vi "lightening arrange.vi"() -> ()   [LabVIEW 2014]
panel:
  in  "panel":T1
  out "result":dbl
  out "result 2":dbl
  out "Total elecFee":dbl
  out "Group 1":bool[](array[boolean])
  out "Group 2":bool[](array[boolean])
  out "Group 3":bool[](array[boolean])
  out "NO.":i32
  out "Waveform Graph 2":dbl[][](graph)
  out "Waveform Graph":dbl[](graph)
  out "size(s)":i32
  in  "group 3 power consume (W)":dbl format="%#_13g"
  in  "group 3 Lightening period":i32
  in  "group 2 power consume (W)":dbl format="%#_13g"
  in  "group 2 Lightening period":i32
  in  "group 1 power consume (W)":dbl format="%#_13g"
  in  "group 1 Lightening period":i32
  in  "input envTemp. & elecFee":cluster{"Temp.":dbl[], "elecFee":dbl[]}={"Temp."=[29.6, 26.5, 26.8, 26.8, 26.5, 26.9, 27.8, 28.5, 26.3, 30.1, 33.3, 33.4, 33.9, 32.2, 32.7, 32.7, 32.4, 31.5, 30.5, 29.7, 28.3, 28.2, 27.9, 27.5], "elecFee"=[2.2, 2.2, 2.2, 2.2, 2.2, 2.2, 2.2, 2.2, 3.5, 3.5, 3.5, 3.5, 3.5, 3.5, 3.5, 3.5, 3.5, 3.5, 3.5, 3.5, 3.5, 3.5, 2.2, 2.2]}
  in  "input Parameter":T2={"input COP of ACs"=3.0, "input setDay Temp"=22.0, "input setNight Temp."=20.0}
  # "0~1"
  # "1~2"
  # "2~3"
  # "3~4"
  # "4~5"
  # "5~6"
  # "6~7"
  # "7~8"
  # "8~98~9"
  # "9~10"
  # "10~11"
  # "11~12"
  # "12~13"
  # "13~14"
  # "14~15"
  # "15~16"
  # "16~17"
  # "17~18"
  # "18~19"
  # "19~20"
  # "21~21"
  # "21~22"
  # "22~23"
  # "23~24"
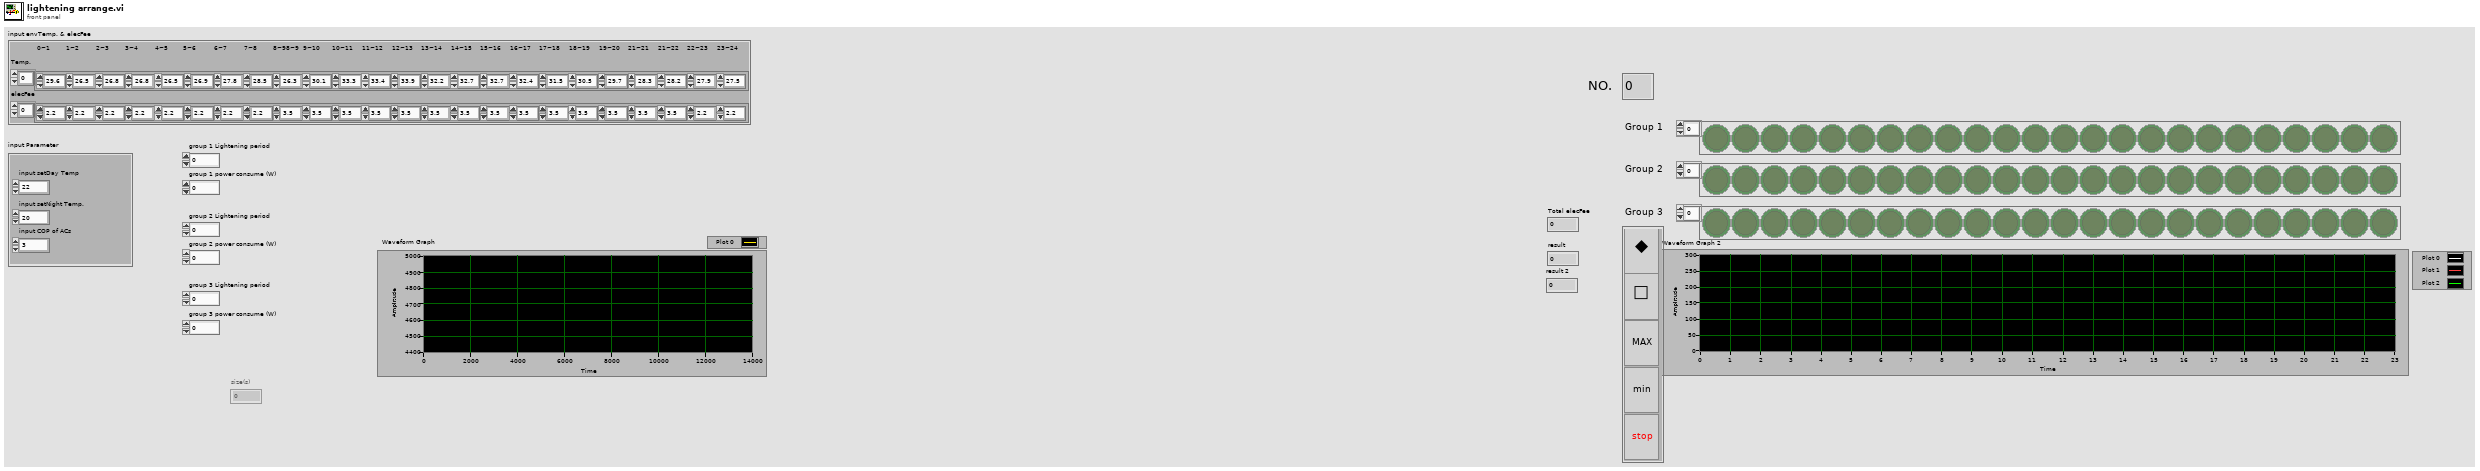
[diagram p1: front panel]
types:
  T1 = cluster{"◆":bool, "□":bool, "MAX":bool, "min":bool, "stop":bool}
  T2 = cluster{"input COP of ACs":dbl, "input setDay Temp":dbl, "input setNight Temp.":dbl}
  T3 = cluster{"group Outcome":cluster{"Lightening Schedule":bool[], "group hourly total elecFee":dbl[], "group Total elecFee":dbl, "group hourly ACs elecFee":dbl[], "group ACs elecFee":dbl, "group hourly LEDs elecFee":dbl[], "group Total LEDs elecFee":dbl}, "group Outcome 2":cluster{"Lightening Schedule":bool[], "group hourly total elecFee":dbl[], "group Total elecFee":dbl, "group hourly ACs elecFee":dbl[], "group ACs elecFee":dbl, "group hourly LEDs elecFee":dbl[], "group Total LEDs elecFee":dbl}, "group Outcome 3":cluster{"Lightening Schedule":bool[], "group hourly total elecFee":dbl[], "group Total elecFee":dbl, "group hourly ACs elecFee":dbl[], "group ACs elecFee":dbl, "group hourly LEDs elecFee":dbl[], "group Total LEDs elecFee":dbl}, "Total elecFee":dbl}[]
  T4 = cluster{"group Outcome":cluster{"Lightening Schedule":bool[], "group hourly total elecFee":dbl[], "group Total elecFee":dbl, "group hourly ACs elecFee":dbl[], "group ACs elecFee":dbl, "group hourly LEDs elecFee":dbl[], "group Total LEDs elecFee":dbl}, "group Outcome 2":cluster{"Lightening Schedule":bool[], "group hourly total elecFee":dbl[], "group Total elecFee":dbl, "group hourly ACs elecFee":dbl[], "group ACs elecFee":dbl, "group hourly LEDs elecFee":dbl[], "group Total LEDs elecFee":dbl}, "group Outcome 3":cluster{"Lightening Schedule":bool[], "group hourly total elecFee":dbl[], "group Total elecFee":dbl, "group hourly ACs elecFee":dbl[], "group ACs elecFee":dbl, "group hourly LEDs elecFee":dbl[], "group Total LEDs elecFee":dbl}, "Total elecFee":dbl}
  T5 = cluster{"Lightening Schedule":bool[], "group hourly total elecFee":dbl[], "group Total elecFee":dbl, "group hourly ACs elecFee":dbl[], "group ACs elecFee":dbl, "group hourly LEDs elecFee":dbl[], "group Total LEDs elecFee":dbl}
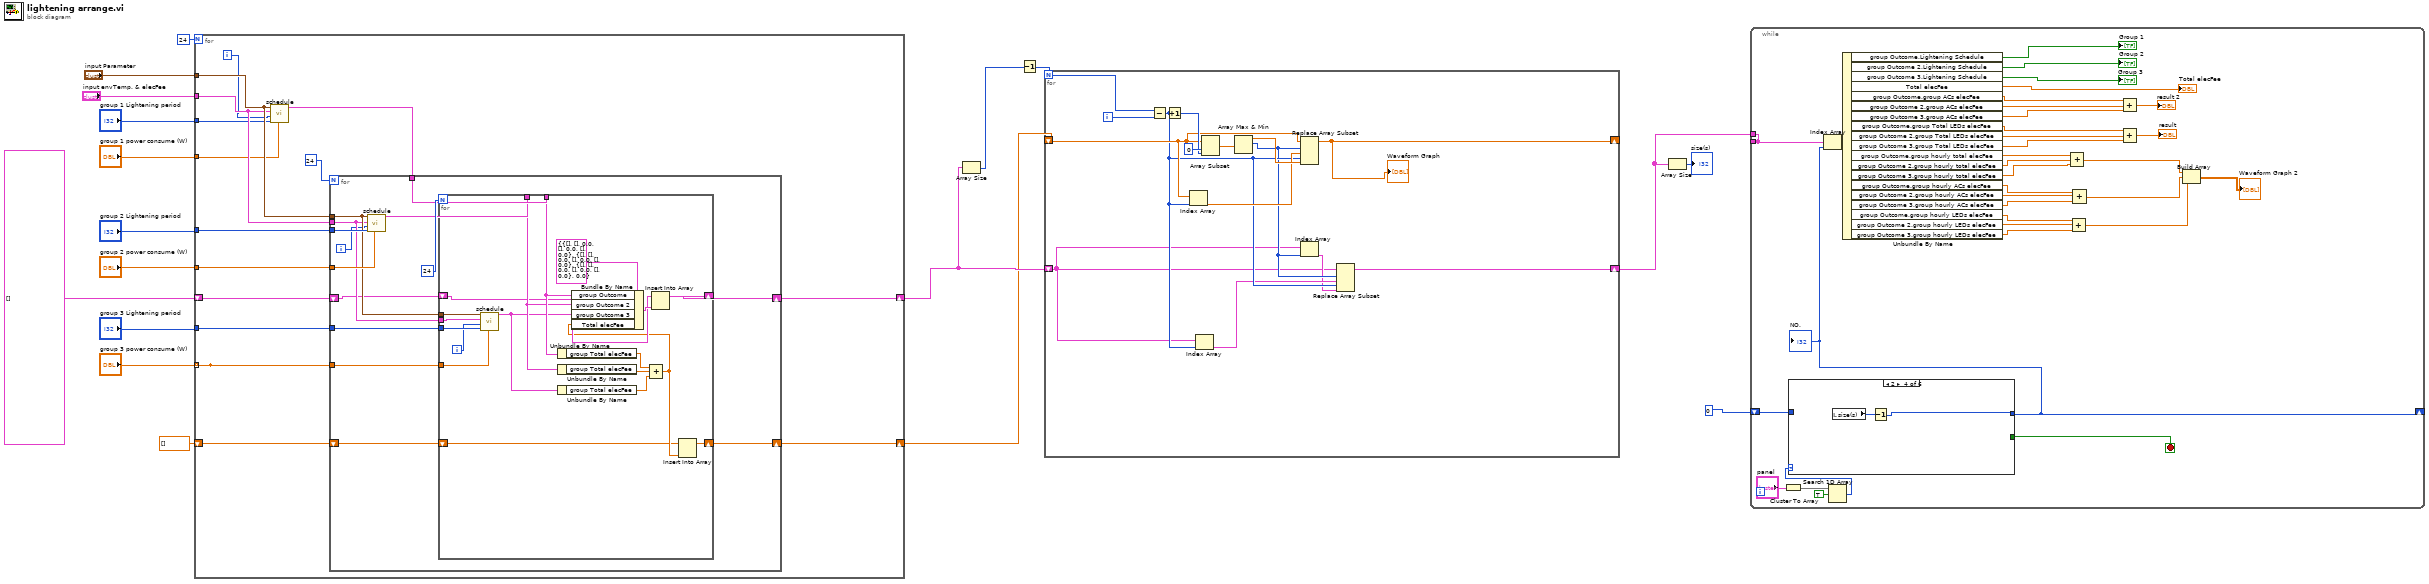
[diagram p0: block diagram]
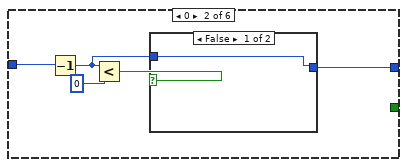
[diagram p3: hidden frame]
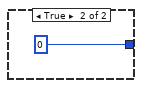
[diagram p4: hidden frame]
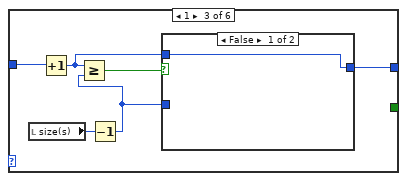
[diagram p5: hidden frame]
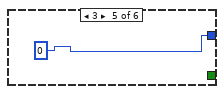
[diagram p7: hidden frame]
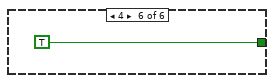
[diagram p8: hidden frame]
diagram:
  n1 = for {
    N: 24 -> [_]
    tunnel: "input Parameter" -> [w32]
    tunnel: "input envTemp. & elecFee" -> [w31]
    tunnel: "group 1 Lightening period" -> [w30]
    tunnel: "group 1 power consume (W)" -> [w29]
    tunnel: "group 2 Lightening period" -> [w28]
    tunnel: "group 2 power consume (W)" -> [w27]
    tunnel: "group 3 Lightening period" -> [w25]
    tunnel: "group 3 power consume (W)" -> [w24]
    tunnel: [w24] -> _ mode=indexing
    shift-right: [w21] -> w8
    shift-left: T3 [] -> [w22]
    shift-right: [w20] -> w5
    shift-left: dbl[] [] -> [w19]
    i -> [w23]
    n2 = call "schedule.vi"("Lighting Power Consume (W)"=w29, "Lenght of Light Period (hr)"=w30, "Start Time of Light Period"=w23, "input envTemp. & elecFee"=w31, "input Parameter"=w32) -> ("group Outcome"=w26:T5)  [unwired: 6 in]
    n3 = for {
      N: 24 -> [_]
      tunnel: w32 -> [w42]
      tunnel: w31 -> [w41]
      tunnel: w28 -> [w47]
      tunnel: w27 -> [w46]
      tunnel: w26 -> [w44]
      tunnel: w25 -> [w40]
      tunnel: w24 -> [w39]
      shift-right: [w37] -> w21
      shift-left: w22 -> [w36]
      shift-right: [w35] -> w20
      shift-left: w19 -> [w34]
      i -> [w38]
      n4 = call "schedule.vi"("Lighting Power Consume (W)"=w46, "Lenght of Light Period (hr)"=w47, "Start Time of Light Period"=w38, "input envTemp. & elecFee"=w41, "input Parameter"=w42) -> ("group Outcome"=w43:T5)  [unwired: 6 in]
      n5 = for {
        N: 24 -> [_]
        tunnel: w44 -> [w57]
        tunnel: w43 -> [w56]
        tunnel: w42 -> [w65]
        tunnel: w41 -> [w64]
        tunnel: w40 -> [w63]
        tunnel: w39 -> [w62]
        shift-right: [w53] -> w37
        shift-left: w36 -> [w52]
        shift-right: [w50] -> w35
        shift-left: w34 -> [w49]
        i -> [w61]
        n6 = call "schedule.vi"("Lighting Power Consume (W)"=w62, "Lenght of Light Period (hr)"=w63, "Start Time of Light Period"=w61, "input envTemp. & elecFee"=w64, "input Parameter"=w65) -> ("group Outcome"=w55:T5)  [unwired: 6 in]
        n7 = Unbundle By Name(w57) -> ("group Total elecFee"=w60:dbl)
        n8 = Unbundle By Name(w56) -> ("group Total elecFee"=w59:dbl)
        n9 = Unbundle By Name(w55) -> ("group Total elecFee"=w58:dbl)
        n10 = Compound Arithmetic op=ADD(w60, w59, w58) -> (w51:dbl)
        n11 = Bundle By Name(cluster=T4 {"group Outcome"={"Lightening Schedule"=[], "group hourly total elecFee"=[], "group Total elecFee"=0.0, "group hourly ACs elecFee"=[], "group ACs elecFee"=0.0, "group hourly LEDs elecFee"=[], "group Total LEDs elecFee"=0.0}, "group Outcome 2"={"Lightening Schedule"=[], "group hourly total elecFee"=[], "group Total elecFee"=0.0, "group hourly ACs elecFee"=[], "group ACs elecFee"=0.0, "group hourly LEDs elecFee"=[], "group Total LEDs elecFee"=0.0}, "group Outcome 3"={"Lightening Schedule"=[], "group hourly total elecFee"=[], "group Total elecFee"=0.0, "group hourly ACs elecFee"=[], "group ACs elecFee"=0.0, "group hourly LEDs elecFee"=[], "group Total LEDs elecFee"=0.0}, "Total elecFee"=0.0} ("Cluster"), "group Outcome"=w57, "group Outcome 2"=w56, "group Outcome 3"=w55, "Total elecFee"=w51) -> (w54:T4)
        n12 = Insert Into Array(array=w52, new element=w54) -> (w53:T3)  [unwired: 1 in]
        n13 = Insert Into Array(array=w49, new element=w51) -> (w50:dbl[])  [unwired: 1 in]
      }
    }
  }
  n14 = Array Size(array=w8) -> (size(s)=w9:i32)
  n15 = Decrement(x=w9) -> (x-1=w6:i32)
  n16 = for {
    N: w6 -> [w74]
    shift-right: [w66] -> w2
    shift-left: w8 -> [w67]
    shift-right: [w72] -> _
    shift-left: w5 -> [w73]
    i -> [w75]
    n17 = Subtract(x=w74, y=w75) -> (x-y=w71:i32)
    n18 = Increment(x=w71) -> (x+1=w77:i32)
    n19 = Index Array(array=w73, index=w71) -> (element=w76:dbl)
    n20 = Index Array(array=w67, index=w71) -> (element=w70:T4)
    n21 = Array Subset(array=w73, index=0, length=w77) -> (w79:dbl[])
    n22 = Array Max & Min(array=w79) -> (max value=w78:dbl, max index (indices)=w69:i32)  [unwired: 2 out]
    n23 = Replace Array Subset(array=w73, new element #1=w76, index #1=w69, new element #2=w78, index #2=w71) -> (w72:dbl[])
    "Waveform Graph" <- w72
    n24 = Index Array(array=w67, index=w69) -> (element=w68:T4)
    n25 = Replace Array Subset(array=w67, new element #1=w70, index #1=w69, new element #2=w68, index #2=w71) -> (w66:T3)
  }
  n26 = Array Size(array=w2) -> (size(s)=→"size(s)":i32)
  n27 = while {
    tunnel: [w81] -> _
    shift-right: [w109] -> _
    shift-left: 0 -> [w110]
    tunnel: w2 -> [w81]
    stop <- w95 stop-if-true
    n28 = Cluster To Array(cluster="panel") -> (array=w113:bool[])
    n29 = Search 1D Array(1D array=w113, element=TRUE) -> (index of element=w111:i32)  [unwired: 1 in]
    n30 = case shown="2" w111 {
      tunnel: w110 -> [w115 w120 w128 _ _ _]
      tunnel: [w115 w117 w124 w131 0 _] -> w109
      tunnel: [_ _ _ _ _ TRUE] -> w95
      frame -1, Default {
      }
      frame 0 {
        n31 = Decrement(x=w120) -> (x-1=w116:i32)
        n32 = Less?(x=w116, y=0) -> (x < y?=w118:bool)
        n33 = case shown="False" w118 {
          tunnel: [w121 0 ("y")] -> w117
          tunnel: w116 -> [w121 _]
          frame False {
          }
          frame True {
          }
        }
      }
      frame 1 {
        n34 = local read "size(s)"() -> (w127:i32)
        n35 = Increment(x=w128) -> (x+1=w123:i32)
        n36 = Decrement(x=w127) -> (x-1=w125:i32)
        n37 = Greater Or Equal?(x=w123, y=w125) -> (x >= y?=w126:bool)
        n38 = case shown="False" w126 {
          tunnel: w125 -> [_ w130]
          tunnel: [w129 w130] -> w124
          tunnel: w123 -> [w129 _]
          frame False {
          }
          frame True {
          }
        }
      }
      frame 2 {
        n39 = local read "size(s)"() -> (w132:i32)
        n40 = Decrement(x=w132) -> (x-1=w131:i32)
      }
      frame 3 {
      }
      frame 4 {
      }
    }
    "NO." <- w109
    n41 = Index Array(array=w81, index=w109) -> (element=w108:T4)
    n42 = Unbundle By Name(w108) -> ("group Outcome.Lightening Schedule"=→"Group 1":bool[], "group Outcome 2.Lightening Schedule"=→"Group 2":bool[], "group Outcome 3.Lightening Schedule"=→"Group 3":bool[], "Total elecFee"=→"Total elecFee":dbl, "group Outcome.group ACs elecFee"=w107:dbl, "group Outcome 2.group ACs elecFee"=w106:dbl, "group Outcome 3.group ACs elecFee"=w105:dbl, "group Outcome.group Total LEDs elecFee"=w104:dbl, "group Outcome 2.group Total LEDs elecFee"=w103:dbl, "group Outcome 3.group Total LEDs elecFee"=w102:dbl, "group Outcome.group hourly total elecFee"=w94:dbl[], "group Outcome 2.group hourly total elecFee"=w93:dbl[], "group Outcome 3.group hourly total elecFee"=w92:dbl[], "group Outcome.group hourly ACs elecFee"=w91:dbl[], "group Outcome 2.group hourly ACs elecFee"=w90:dbl[], "group Outcome 3.group hourly ACs elecFee"=w89:dbl[], "group Outcome.group hourly LEDs elecFee"=w88:dbl[], "group Outcome 2.group hourly LEDs elecFee"=w87:dbl[], "group Outcome 3.group hourly LEDs elecFee"=w86:dbl[])
    n43 = Compound Arithmetic op=ADD(w94, w93, w92) -> (w85:dbl[])
    n44 = Compound Arithmetic op=ADD(w88, w87, w86) -> (w82:dbl[])
    n45 = Compound Arithmetic op=ADD(w91, w90, w89) -> (w83:dbl[])
    n46 = Compound Arithmetic op=ADD(w107, w106, w105) -> (→"result 2":dbl)
    n47 = Compound Arithmetic op=ADD(w104, w103, w102) -> (→"result":dbl)
    n48 = Build Array(w85, w83, w82) -> (→"Waveform Graph 2":dbl[][])
  }
